vi "GyropMoveFunc.vi"(8 "error in (no error)":errorcluster, 11 "期望旋转角度":dbl format="%.2f") -> (0 "error out":errorcluster)   [LabVIEW 2017]
uses:
  <vilib>/Platform/TimedLoop/XDataNode/timing_clust.ctl
  <vilib>/Platform/TimedLoop/XDataNode/nitl_modes.ctl
  <vilib>/Platform/TimedLoop/XDataNode/wakeup.ctl
  <vilib>/myRIO/Common/Instrument Driver Framework/myRIO v1.0/I2C/vis/myRIO v1.0 Close I2C.vi
  <vilib>/myRIO/Common/Instrument Driver Framework/myRIO v1.0/I2C/vis/myRIO v1.0 Unreserve I2C.vi
  <vilib>/myRIO/Common/Instrument Driver Framework/myRIO v1.0/I2C/vis/myRIO v1.0 Build MUX Configuration I2C.vi
  <vilib>/myRIO/Common/Instrument Driver Framework/myRIO v1.0/Resource Manager/vis/myRIO v1.0 Unreserve Channel List.vi
  <vilib>/myRIO/Common/Instrument Driver Framework/myRIO v1.0/Resource Manager/vis/myRIO v1.0 Create Configuration List.vi
  <vilib>/myRIO/Common/Instrument Driver Framework/myRIO v1.0/Resource Manager/vis/myRIO v1.0 Unreserve Channel.vi
  <vilib>/myRIO/Common/Instrument Driver Framework/myRIO v1.0/Resource Manager/vis/myRIO v1.0 Build Mutex Name.vi
  <vilib>/addons/control/pid/pid.llb/PID (DBL).vi
  <vilib>/Utility/error.llb/Error Cluster From Error Code.vi
  <vilib>/myRIO/Common/Instrument Driver Framework/myRIO v1.0/I2C/vis/myRIO v1.0 Shutdown I2C.vi
  <vilib>/myRIO/Common/Instrument Driver Framework/myRIO v1.0/Resource Manager/vis/myRIO v1.0 Configure IO.vi
  <vilib>/myRIO/Common/Instrument Driver Framework/Utilities/vis/Configuration Manager.vi
  <vilib>/myRIO/Common/Instrument Driver Framework/Utilities/vis/IO Manager.vi
  <vilib>/myRIO/Common/Instrument Driver Framework/myRIO v1.0/myRIO v1.0 Close.vi
  <vilib>/Platform/TimedLoop/XDataNode/XDataNode.xnode
  <vilib>/Platform/TimedLoop/XDataNode/XDNodeRunTimeDep.lvlib
  <vilib>/addons/control/pid/NI_PID_pid.lvlib
  <vilib>/myRIO/Instrument Drivers/Onboard IO/I2C/I2C.lvlib
panel:
  out "角度比较":cluster{"期望旋转角度":dbl, "转动的角度":dbl}(graph)
  out "实际转动的角度":dbl caption="转动的角度" format="%0.2f"
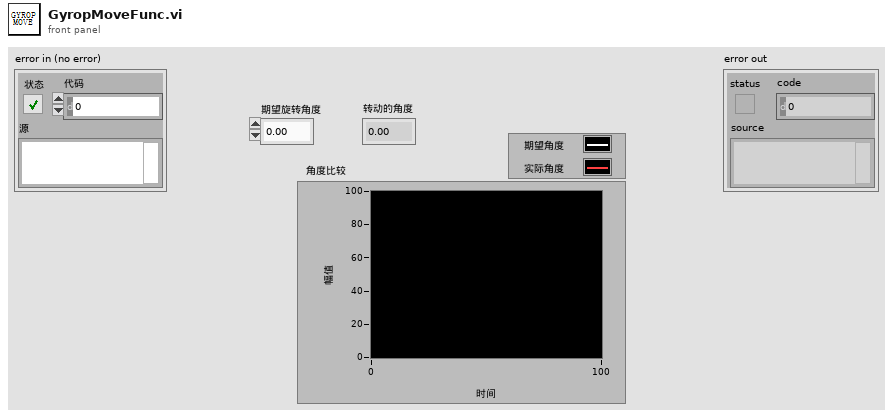
[diagram p1: front panel]
types:
  T1 = typedef "I2C.lvlib/I2C Reference.ctl" = cluster{"myRIO Reference":T2, "I2C Channels Enum":T6, "I2C Configuration":T7}
  T2 = typedef "myRIO Generic Hardware Reference.ctl" = cluster{"myRIO Model":T3, "myRIO Hardware Reference":T4}
  T3 = typedef "Hardware Version Enum.ctl" = enum16{"Unknown", "myRIO-1900", "myRIO-1950", "roboRIO", "NI ELVIS RIO CM"}
  T4 = typedef "myRIO v1.0 Reference.ctl" = cluster{"Generic FPGA Reference":T5, "Allow multiple opens":bool}
  T5 = typedef "Generic FPGA Reference.ctl" = refnum<k20>
  T6 = typedef "I2C Channels Enum.ctl" = enum16{"Not Connected", "A/I2C", "B/I2C", "I2C/I2C"}
  T7 = typedef "I2C.lvlib/I2C Configuration.ctl" = cluster{"I2C Transfer Rate":T8}
  T8 = typedef "I2C.lvlib/I2C Transfer Rate.ctl" = enum16{"Standard mode (100 kbps)", "Fast mode (400 kbps)"}
  T9 = typedef "XDNodeRunTimeDep.lvlib/timing_clust.ctl" = cluster{"Expected End [f-1]":u64, "Actual End [f-1]":u64, "Finished Late? [f-1]":bool, "Expected End [i-1]":u64, "Actual End [i-1]":u64, "Finished Late? [i-1]":bool, "Expected Start [i]":u64, "Actual Start [i]":u64, "Expected Start [f]":u64, "Actual Start [f]":u64, "Source Name":string, "Structure Name":string, "Period":i64, "Deadline":i64, "Offset":i64, "Start":i64, "Priority":i32, "Timeout":i32, "Mode":T10, "Wakeup Reason":T11, "Error":errorcluster, "Source Type":string, "Secondary Source Type":string, "Global End Time":u64, "Global Start Time":u64, "Frame Duration":u64, "Iteration Duration":u64, "Assigned CPU":i32, "I/O Scan Engine Mode":u32}
  T10 = typedef "XDNodeRunTimeDep.lvlib/nitl_modes.ctl" = enum32{"No Change", "Process missed periods, maintain original phase", "Discard missed periods, maintain original phase", "Process missed periods, ignore original phase", "Discard missed periods, ignore original phase"}
  T11 = typedef "XDNodeRunTimeDep.lvlib/wakeup.ctl" = enum32{"Normal", "Aborted", "Asynchronous wakeup", "Timing source error", "Timed loop error", "Timeout"}
  T12 = cluster{"proportional gain (Kc)":dbl, "integral time (Ti, min)":dbl, "derivative time (Td, min)":dbl}
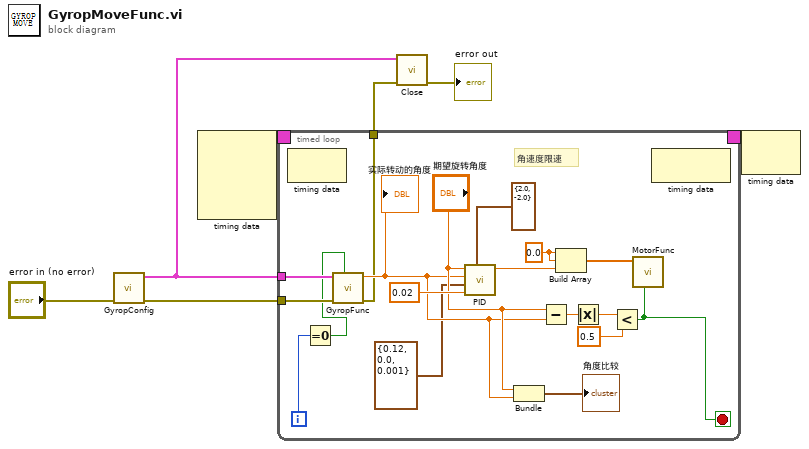
[diagram p0: block diagram]
diagram:
  n1 = call "GyropConfig.vi"("error in (no error)"="error in (no error)") -> ("error out"=w4:errorcluster, "I2C对象的引用"=w1:T1)  [unwired: 9 in]
  n2 = node-c288() -> (w7:T9)  [unwired: 4 in]
  n3 = timed-loop {
    timing: w7 -> [_]
    timing-out: [_] -> w6
    tunnel: w4 -> [w24]
    tunnel: w1 -> [w25]
    tunnel: [w9] -> w3
    i -> [w23]
    stop <- w13 stop-if-true
    w18 = 0.0 ("元素")
    # "角速度限速"
    n4 = node-c288() -> ()  [unwired: 1 in, 1 out]
    n5 = Equal To 0?(x=w23) -> (x = 0?=w22:bool)
    n6 = call "GyropFunc.vi"("重置积分器"=w22, "error in (no error)"=w24, "I2C Ref In"=w25) -> ("error out"=w9:errorcluster, "转动的角度"=w11:dbl)  [unwired: 6 in]
    "实际转动的角度" <- w11
    n7 = call-poly <vilib>:"PID.vi"("output range"=cluster{"output high":dbl, "output low":dbl} {"output high"=2.0, "output low"=-2.0}, "dt (s)"=0.02, "PID gains"=T12 {"proportional gain (Kc)"=0.12, "integral time (Ti, min)"=0.0, "derivative time (Td, min)"=0.001}, "process variable"=w11, "setpoint"="期望旋转角度") -> ("output"=w19:dbl)  [unwired: 5 in, 1 out]
    n8 = Bundle("期望旋转角度"="期望旋转角度", "转动的角度"=w11) -> (→"角度比较":cluster{"期望旋转角度":dbl, "转动的角度":dbl})  [unwired: 1 in]
    n9 = Subtract(x="期望旋转角度", y=w11) -> (x-y=w16:dbl)
    n10 = Build Array(w18, w18, w19) -> (w17:dbl[])
    n11 = Absolute Value(x=w16) -> (abs(x)=w15:dbl)
    n12 = Less?(x=w15, y=0.5) -> (x < y?=w13:bool)
    n13 = call "MotorFunc.vi"("停止"=w13, "把当前坐标系下期望小\n车在X、Y、θ的速度作\n为逆运算的输入"=w17) -> ()  [unwired: 8 in, 2 out]
    n14 = node-c288() -> ()  [unwired: 1 in, 1 out]
  }
  n15 = call <vilib>:"Close.vi"("error in (no error)"=w3, "I2C Ref In"=w1) -> ("error out"=→"error out":errorcluster)  [unwired: 9 in]
  n16 = node-c288(w6) -> ()  [unwired: 1 out]
